vi "get_myMsgEvent.vi"(8 "error in (no error)":errorcluster, 11 "MoAgSy_AgentBase in":refnum<class "MoAgSy_AgentBase.lvclass">) -> (0 "error out":errorcluster, 2 "HGF_BaseClasses.lvlib:HGF_Event.lvclass":refnum<class "HGF_Event.lvclass">, 3 "MoAgSy_AgentBase out":refnum<class "MoAgSy_AgentBase.lvclass">)   [LabVIEW 2009, in "MoAgSy_Base.lvlib" / "MoAgSy_AgentBase.lvclass"]
uses:
  MoAgSy_AgentBase.lvclass
  HGF_BaseClasses/HGF_Event/HGF_Event.lvclass
  MoAgSy_AgentBase.lvclass/MoAgSy_AgentBase.ctl
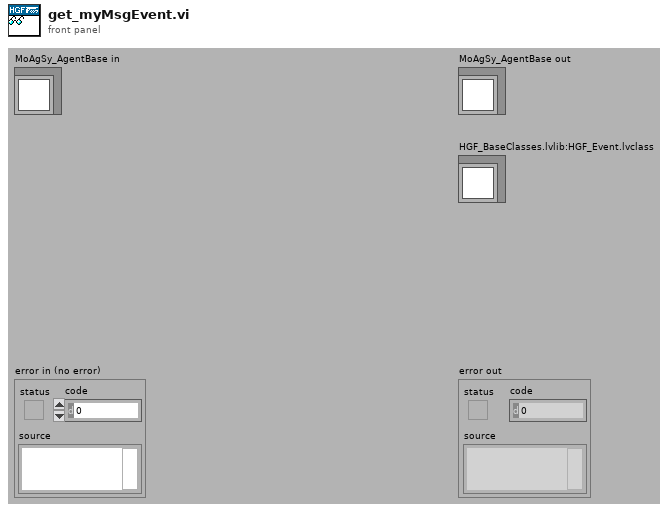
[diagram p1: front panel]
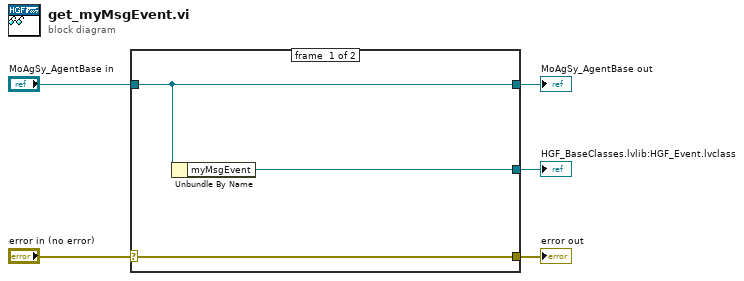
[diagram p0: block diagram]
diagram:
  n1 = case shown="No Error" "error in (no error)" {
    selector: "error in (no error)" -> [w8 w9]
    tunnel: [w8 w9] -> w4
    tunnel: [w7 w10] -> w2
    tunnel: "MoAgSy_AgentBase in" -> [w7 w10]
    tunnel: [w6 _] -> w1
    frame #0 {
      n2 = Unbundle By Name(w7) -> ("myMsgEvent"=w6:refnum<class "HGF_Event.lvclass">)
    }
    frame #1 {
    }
  }
  "error out" <- w4
  "MoAgSy_AgentBase out" <- w2
  "HGF_BaseClasses.lvlib:HGF_Event.lvclass" <- w1
